vi "QueryServer_SetStreamAnalogInputData.vi"(6 "error in (no error)":errorcluster, 8 "AnalogInputData":T1, 9 "gRPCid":T2) -> (0 "error out":errorcluster, 3 "gRPCid out":T2)   [LabVIEW 2019, in "labview-grpc-query-server.lvlib"]
uses:
  labview-grpc-query-server.lvlib
  VIs/grpcId.ctl
  QueryServer_AnalogInputData.ctl
  d149c175-cf88-4dc1-b2b5-9725cea78de2.vi
  VIs/gprc-support.lvlib
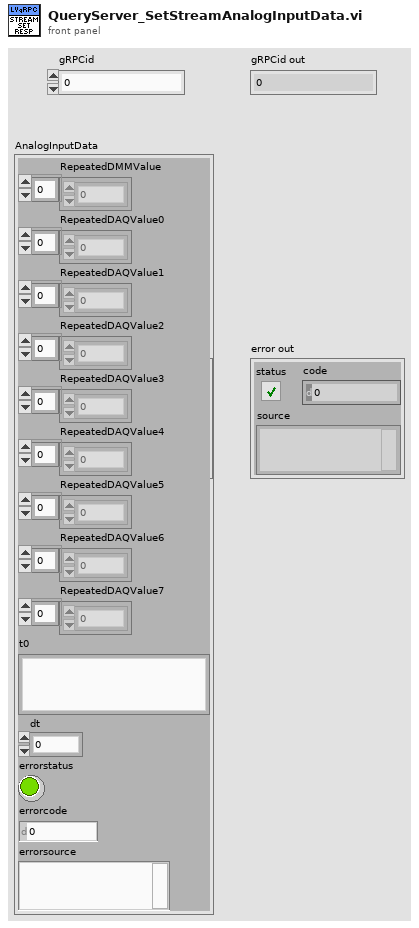
[diagram p1: front panel]
types:
  T1 = typedef "labview-grpc-query-server.lvlib/QueryServer_AnalogInputData.ctl" = cluster{"RepeatedDMMValue":dbl[], "RepeatedDAQValue0":dbl[], "RepeatedDAQValue1":dbl[], "RepeatedDAQValue2":dbl[], "RepeatedDAQValue3":dbl[], "RepeatedDAQValue4":dbl[], "RepeatedDAQValue5":dbl[], "RepeatedDAQValue6":dbl[], "RepeatedDAQValue7":dbl[], "t0":string, "dt":dbl, "errorstatus":bool, "errorcode":i32, "errorsource":string}
  T2 = typedef "gprc-support.lvlib/grpcId.ctl" = u64
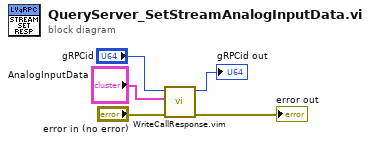
[diagram p0: block diagram]
diagram:
  n1 = call "WriteCallResponse.vim"("error in (no error)"="error in (no error)", "Response Data"="AnalogInputData", "gRPCid in"="gRPCid") -> ("error out"=→"error out":errorcluster, "gRPCid"=→"gRPCid out":T2)  [unwired: 7 in]
